vi "Disconnect from Typedef.vi"(6 "Variant in":variant, 7 "Shift Pressed?":bool, 8 "error in (no error)":errorcluster, 10 "QD Combo Box Ref":refnum<vi>, 11 "QD Launch VI Ref":refnum<vi>) -> (0 "error out":errorcluster, 4 "Variant out":variant)   [LabVIEW 2013]
doc: "Disconnects controls or constants from their source type definition. If [Shift] is also pressed, disconnects all controls/constants within the selection from their source type definitions recursively.\n\nDefault Shortcut - [Y]"
uses:
  <vilib>/Utility/traverseref.llb/TRef TravTarget.ctl
  <vilib>/Utility/traverseref.llb/VI Scripting - Traverse.lvlib
panel:
  in  "Undo Name":string="Disconnect from Typedef"
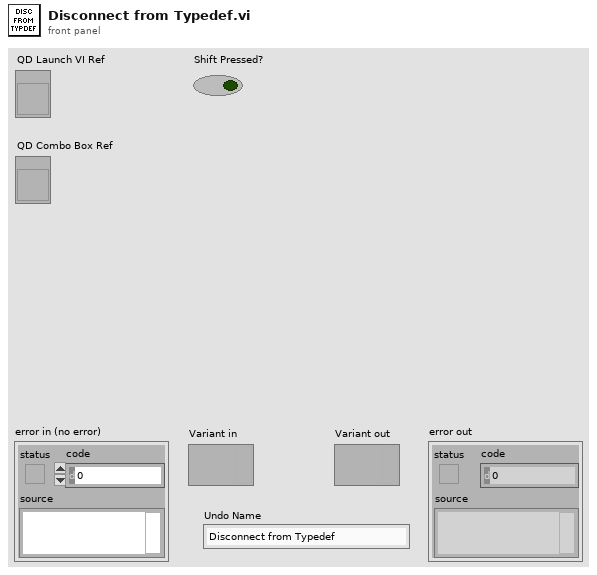
[diagram p1: front panel]
types:
  T1 = typedef "TRef TravTarget.ctl" = enum16{"FP", "BD", "Other"}
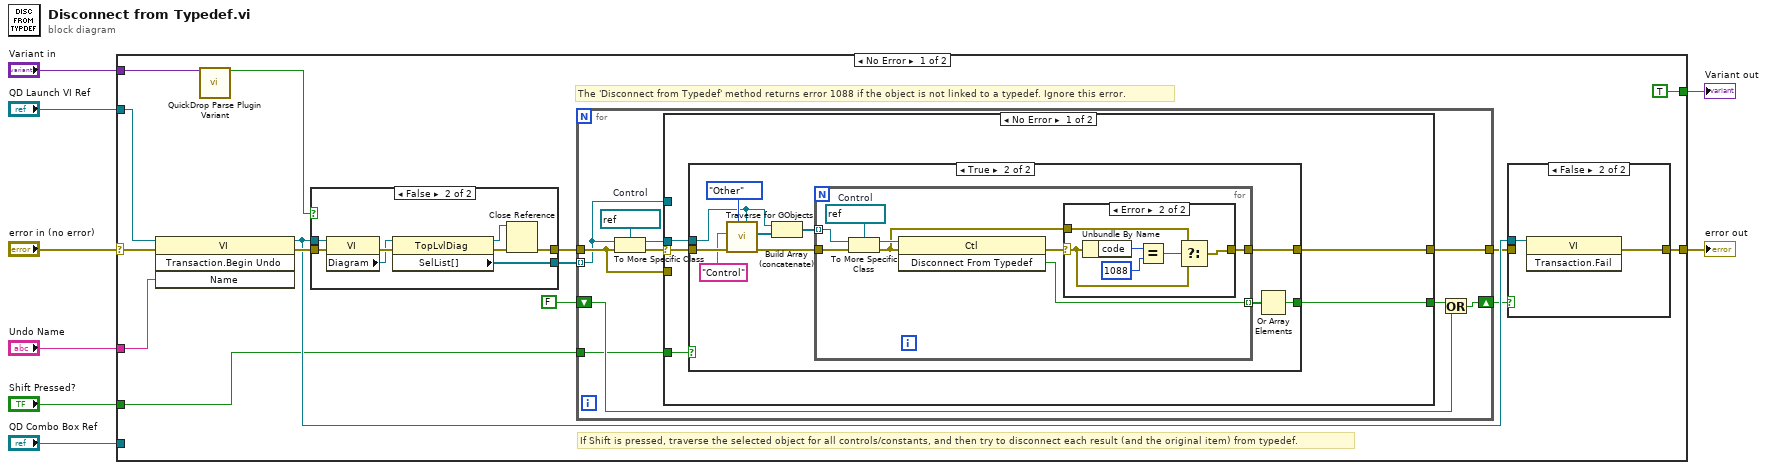
[diagram p0: block diagram]
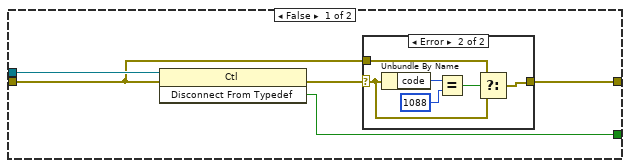
[diagram p2: hidden frame]
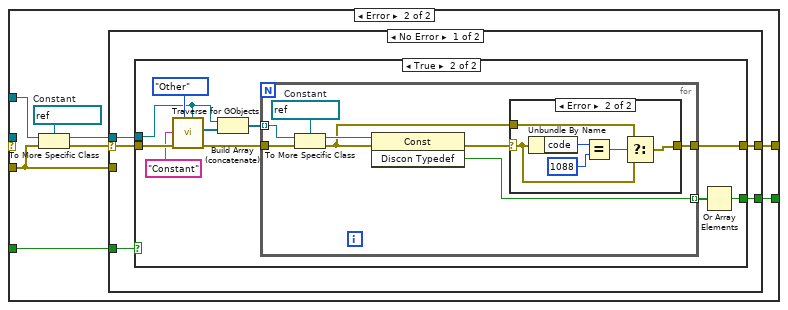
[diagram p5: hidden frame]
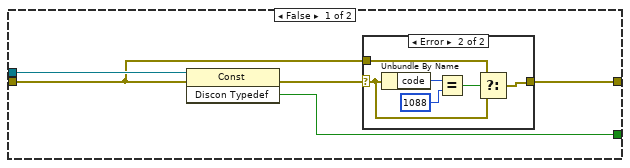
[diagram p6: hidden frame]
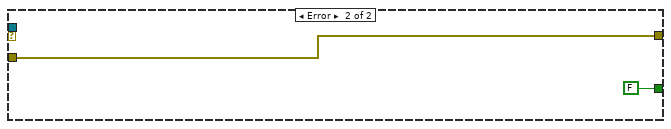
[diagram p9: hidden frame]
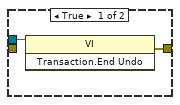
[diagram p10: hidden frame]
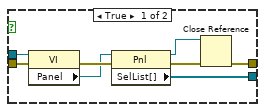
[diagram p11: hidden frame]
diagram:
  n1 = case shown="No Error" "error in (no error)" {
    selector: "error in (no error)" -> [w22 w148]
    tunnel: [w16 w148] -> w7
    tunnel: "QD Launch VI Ref" -> [w21 _]
    tunnel: "Shift Pressed?" -> [w10 _]
    tunnel: "QD Combo Box Ref" -> [_ _]
    tunnel: "Variant in" -> [w23 _]
    tunnel: "Undo Name" -> [w20 _]
    tunnel: [TRUE _] -> w1
    frame No Error {
      # "If Shift is pressed, traverse the selected object for all controls/constants, and then try to disconnect each result (and the original item) from typedef."
      # "The 'Disconnect from Typedef' method returns error 1088 if the object is not linked to a typedef. Ignore this error."
      n2 = invoke class="VI" method="Transaction.Begin Undo"(reference=w21, error in=w22, "Name"=w20) -> (reference out=w14:refnum<vi>, error out=w17:errorcluster)  [unwired: 1 in, 2 out]
      n3 = call <vilib>:"QuickDrop Parse Plugin Variant.vi"("QDKS Variant in"=w23) -> ("QD Launch VI Panel?"=w18:bool)  [unwired: 12 in, 2 out]
      n4 = case shown="False" w18 {
        tunnel: w17 -> [w139 w147]
        tunnel: w14 -> [w138 w146]
        tunnel: [w133 w141] -> w15
        tunnel: [w132 w140] -> w11
        frame True {
          n5 = property class="VI"(reference=w138, error in=w139) -> (error out=w137:errorcluster, "Panel"=w136:refnum<vi>)  [unwired: 1 out]
          n6 = property class="Pnl"(reference=w136, error in=w137) -> (reference out=w134:refnum<vi>, error out=w135:errorcluster, "SelList[]"=w132:refnum<vi>[])
          n7 = Close Reference(reference=w134, error in (no error)=w135) -> (error out=w133:errorcluster)
        }
        frame False {
          n8 = property class="VI"(reference=w146, error in=w147) -> (error out=w145:errorcluster, "Diagram"=w144:refnum<vi>)  [unwired: 1 out]
          n9 = property class="TopLvlDiag"(reference=w144, error in=w145) -> (reference out=w142:refnum<vi>, error out=w143:errorcluster, "SelList[]"=w140:refnum<vi>[])
          n10 = Close Reference(reference=w142, error in (no error)=w143) -> (error out=w141:errorcluster)
        }
      }
      n11 = for {
        shift-right: [w33] -> w12
        shift-left: FALSE -> [w31]
        tunnel: w11 -> [w24] mode=indexing
        tunnel: w15 -> [w25]
        tunnel: [w27] -> w9
        tunnel: w10 -> [w26]
        w32 = refnum<vi> refnum  # Control
        n12 = To More Specific Class(target class=w32, reference=w24, error in=w25) -> (specific class reference=w29:refnum<vi>, error out=w30:errorcluster)
        n13 = case shown="No Error" w30 {
          selector: w30 -> [w38 _]
          tunnel: w29 -> [w37 _]
          tunnel: [w36 w77] -> w28
          tunnel: [w35 w79] -> w27
          tunnel: w26 -> [w34 w76]
          tunnel: w25 -> [_ w78]
          tunnel: w24 -> [_ w83]
          frame No Error {
            n14 = case shown="True" w34 {
              tunnel: w38 -> [w40 w58]
              tunnel: w37 -> [w43 w53]
              tunnel: [w42 w51] -> w36
              tunnel: [w39 w59] -> w35
              frame False {
                n15 = invoke class="Ctl" method="Disconnect From Typedef"(reference=w43, error in=w40) -> (error out=w41:errorcluster, "Discon Typedef"=w42:bool)  [unwired: 1 in, 1 out]
                n16 = case shown="Error" w41 {
                  selector: w41 -> [w44 w47]
                  tunnel: [w44 w46] -> w39
                  tunnel: w40 -> [_ w45]
                  frame No Error {
                  }
                  frame Error {
                    n17 = Unbundle By Name(w47) -> ("code"=w50:i32)
                    n18 = Equal?(x=w50, y=1088) -> (x = y?=w48:bool)
                    n19 = Select(t=w45, s=w48, f=w47) -> (s? t:f=w46:errorcluster)
                  }
                }
              }
              frame True {
                n20 = call <vilib>:"Traverse for GObjects.vi"("Other Refnum"=w53, "Traverse Target"=TRef_TravTarget."Other", "error in (no error)"=w58, "Class Name"="Control") -> ("error out"=w55:errorcluster, "References"=w54:refnum<vi>[])  [unwired: 4 in, 2 out]
                n21 = Build Array (concatenate)(w53, w54) -> (w52:refnum<vi>[])
                n22 = for {
                  tunnel: [w68] -> w60 mode=indexing
                  tunnel: [w62] -> w59
                  tunnel: w55 -> [w67]
                  tunnel: w52 -> [w66] mode=indexing
                  w65 = refnum<vi> refnum  # Control
                  n23 = To More Specific Class(target class=w65, reference=w66, error in=w67) -> (specific class reference=w64:refnum<vi>, error out=w61:errorcluster)
                  n24 = invoke class="Ctl" method="Disconnect From Typedef"(reference=w64, error in=w61) -> (error out=w63:errorcluster, "Discon Typedef"=w68:bool)  [unwired: 1 in, 1 out]
                  n25 = case shown="Error" w63 {
                    selector: w63 -> [w69 w72]
                    tunnel: [w69 w71] -> w62
                    tunnel: w61 -> [_ w70]
                    frame No Error {
                    }
                    frame Error {
                      n26 = Unbundle By Name(w72) -> ("code"=w75:i32)
                      n27 = Equal?(x=w75, y=1088) -> (x = y?=w73:bool)
                      n28 = Select(t=w70, s=w73, f=w72) -> (s? t:f=w71:errorcluster)
                    }
                  }
                }
                n29 = Or Array Elements(Boolean array=w60) -> (logical OR=w51:bool)
              }
            }
          }
          frame Error {
            w82 = refnum<vi> refnum  # Constant
            n30 = To More Specific Class(target class=w82, reference=w83, error in=w78) -> (specific class reference=w80:refnum<vi>, error out=w81:errorcluster)
            n31 = case shown="No Error" w81 {
              selector: w81 -> [w88 _]
              tunnel: w80 -> [w87 _]
              tunnel: [w85 w127] -> w79
              tunnel: w78 -> [_ w127]
              tunnel: [w84 FALSE] -> w77
              tunnel: w76 -> [w86 _]
              frame No Error {
                n32 = case shown="True" w86 {
                  tunnel: w88 -> [w90 w108]
                  tunnel: w87 -> [w93 w103]
                  tunnel: [w92 w101] -> w84
                  tunnel: [w89 w109] -> w85
                  frame False {
                    n33 = invoke class="Const" method="Discon Typedef"(reference=w93, error in=w90) -> (error out=w91:errorcluster, "Discon Typedef"=w92:bool)  [unwired: 1 in, 1 out]
                    n34 = case shown="Error" w91 {
                      selector: w91 -> [w94 w97]
                      tunnel: [w94 w96] -> w89
                      tunnel: w90 -> [_ w95]
                      frame No Error {
                      }
                      frame Error {
                        n35 = Unbundle By Name(w97) -> ("code"=w100:i32)
                        n36 = Equal?(x=w100, y=1088) -> (x = y?=w98:bool)
                        n37 = Select(t=w95, s=w98, f=w97) -> (s? t:f=w96:errorcluster)
                      }
                    }
                  }
                  frame True {
                    n38 = call <vilib>:"Traverse for GObjects.vi"("Other Refnum"=w103, "Traverse Target"=TRef_TravTarget."Other", "error in (no error)"=w108, "Class Name"="Constant") -> ("error out"=w105:errorcluster, "References"=w104:refnum<vi>[])  [unwired: 4 in, 2 out]
                    n39 = Build Array (concatenate)(w103, w104) -> (w102:refnum<vi>[])
                    n40 = for {
                      tunnel: [w118] -> w110 mode=indexing
                      tunnel: [w112] -> w109
                      tunnel: w105 -> [w117]
                      tunnel: w102 -> [w116] mode=indexing
                      w115 = refnum<vi> refnum  # Constant
                      n41 = To More Specific Class(target class=w115, reference=w116, error in=w117) -> (specific class reference=w114:refnum<vi>, error out=w111:errorcluster)
                      n42 = invoke class="Const" method="Discon Typedef"(reference=w114, error in=w111) -> (error out=w113:errorcluster, "Discon Typedef"=w118:bool)  [unwired: 1 in, 1 out]
                      n43 = case shown="Error" w113 {
                        selector: w113 -> [w119 w122]
                        tunnel: [w119 w121] -> w112
                        tunnel: w111 -> [_ w120]
                        frame No Error {
                        }
                        frame Error {
                          n44 = Unbundle By Name(w122) -> ("code"=w125:i32)
                          n45 = Equal?(x=w125, y=1088) -> (x = y?=w123:bool)
                          n46 = Select(t=w120, s=w123, f=w122) -> (s? t:f=w121:errorcluster)
                        }
                      }
                    }
                    n47 = Or Array Elements(Boolean array=w110) -> (logical OR=w101:bool)
                  }
                }
              }
              frame Error {
              }
            }
          }
        }
        n48 = Or(x=w28, y=w31) -> (x .or. y?=w33:bool)
      }
      n49 = case shown="False" w12 {
        tunnel: w14 -> [w128 w130]
        tunnel: [w129 w131] -> w16
        tunnel: w9 -> [_ _]
        frame True {
          n50 = invoke class="VI" method="Transaction.End Undo"(reference=w128) -> (error out=w129:errorcluster)  [unwired: 2 in, 2 out]
        }
        frame False {
          n51 = invoke class="VI" method="Transaction.Fail"(reference=w130) -> (error out=w131:errorcluster)  [unwired: 2 in, 2 out]
        }
      }
    }
    frame Error {
    }
  }
  "error out" <- w7
  "Variant out" <- w1
